vi "EXA_Get_ACPR.vi"(8 "error in":errorcluster, 11 "VISA resource name":refnum<visa-resource-name>) -> (0 "error out":errorcluster, 1 "ACP Sorted":dbl[](array[numeric]), 2 "ACP Values":dbl[](array[numeric]), 3 "VISA resource name":refnum<visa-resource-name>)   [LabVIEW 2016]
panel:
  out "read buffer":string
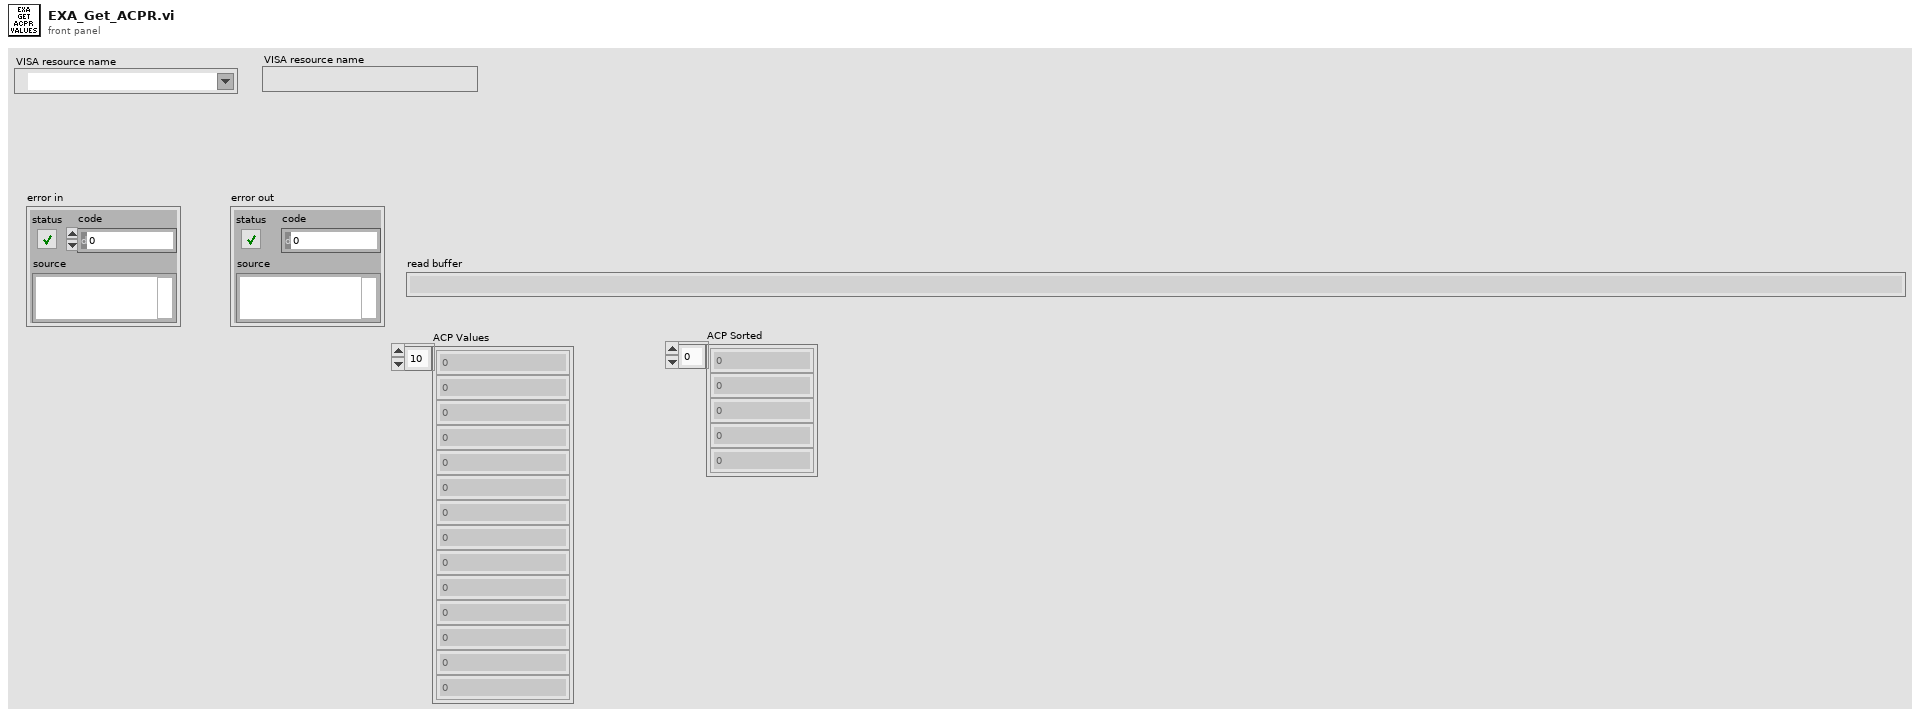
[diagram p1: front panel]
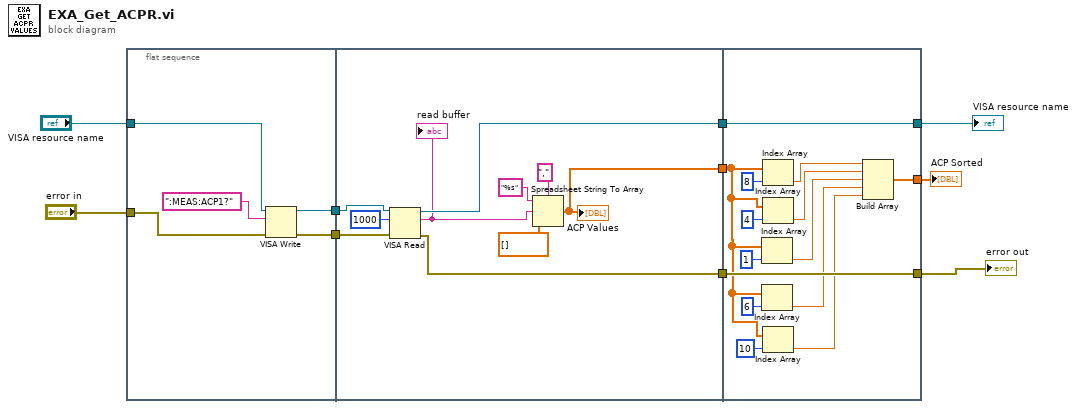
[diagram p0: block diagram]
diagram:
  n1 = flat-sequence {
    tunnel: [w15] -> w10
    tunnel: [w14] -> w9
    tunnel: "VISA resource name" -> [w13]
    tunnel: "error in" -> [w11]
    tunnel: w10 -> [w23]
    tunnel: w9 -> [w24]
    tunnel: [w22] -> w4
    tunnel: [w21] -> w3
    tunnel: [w16] -> w2
    tunnel: [w38] -> w7
    tunnel: [w39] -> w8
    tunnel: w4 -> [w39]
    tunnel: w3 -> [w38]
    tunnel: w2 -> [w32]
    tunnel: [w26] -> w1
    frame #0 {
      n2 = VISA Write(VISA resource name=w13, write buffer=":MEAS:ACP1?" ("format string"), error in (no error)=w11) -> (VISA resource name out=w14:refnum<visa-resource-name>, error out=w15:errorcluster)  [unwired: 1 out]
    }
    frame #1 {
      n3 = VISA Read(VISA resource name=w24, byte count=u32 1000, error in (no error)=w23) -> (VISA resource name out=w22:refnum<visa-resource-name>, read buffer=w17:string, error out=w21:errorcluster)  [unwired: 1 out]
      "read buffer" <- w17
      n4 = Spreadsheet String To Array(delimiter (Tab)=",", format string="%s", spreadsheet string=w17, array type (2D Dbl)=dbl[] []) -> (array=w16:dbl[])
      "ACP Values" <- w16
    }
    frame #2 {
      n5 = Index Array(array=w32, index=1) -> (element=w29:dbl)
      n6 = Index Array(array=w32, index=6) -> (element=w28:dbl)
      n7 = Index Array(array=w32, index=8) -> (element=w31:dbl)
      n8 = Index Array(array=w32, index=4) -> (element=w30:dbl)
      n9 = Index Array(array=w32, index=10) -> (element=w27:dbl)
      n10 = Build Array(w31, w30, w29, w28, w27) -> (w26:dbl[])
    }
  }
  "error out" <- w7
  "VISA resource name" <- w8
  "ACP Sorted" <- w1
